vi "test_fpga.vi"() -> ()   [LabVIEW 2014, in "SYSID.lvlib"]
doc: "This VI was generated automatically using the FPGA Wizard. You can modify the VI normally."
uses:
  SYSID.lvlib
  <vilib>/Platform/TimedLoop/XDataNode/timing_clust.ctl
  <vilib>/Platform/TimedLoop/XDataNode/nitl_modes.ctl
  <vilib>/Platform/TimedLoop/XDataNode/wakeup.ctl
  <vilib>/rvi/Emulation/niFpgaGetClockAttributes.vi
  <vilib>/rvi/Emulation/niFpgaSctlEmulationGetInTimedLoop.vi
  <vilib>/rvi/Emulation/niFpgaEmulationReportErrorSimple.vi
  <vilib>/rvi/Emulation/niFpgaProcessEmulError.vi
  <vilib>/rvi/eio/common/nirviEmuTemplateMethod_errors.vi
  <vilib>/rvi/Emulation/niFpgaCriticalErrorInLSC.vi
  <vilib>/eio/EIONode/EIONode.xnode
  <vilib>/Platform/TimedLoop/XDataNode/XDataNode.xnode
  <vilib>/Platform/TimedLoop/XDataNode/XDNodeRunTimeDep.lvlib
panel:
  out "velocity":sgl
  out "Pendulum Position":i32
  out "_Pendulum Position":i32
  in  "Pendulum Reset":bool
  out "Right Limit":bool
  out "Left Limit":bool
  in  "Brake":bool=TRUE
  in  "Amp Reset":bool=TRUE
  in  "Amp Enable":bool
  out "quad saved (Port0/DIO0,Port0/DIO1)":cluster{"Position":i32, "Index Count":u16}
  out "Stage Position":i32
  out "_quad pos (Port0/DIO0,Port0/DIO1)":i32
  in  "quad reset (Port0/DIO0,Port0/DIO1)":bool
  out "_quad saved (Port0/DIO0,Port0/DIO1)":cluster{"Position":i32, "Index Count":u16}
  in  "AO (ModB/AO2)":fxp<+/-,20,5>
  in  "Drive Command":fxp<+/-,20,5>
  out "AI (ModA/AI0)":fxp<+/-,26,5> format="%.6g"
  in  "Local Stop 0":bool
  out "Actual Loop Rate (Ticks)":u32
  out "Late? Latched":bool
  in  "Loop Rate (Ticks)":u32=571
  in  "Reset":bool
  in  "Start 0":bool
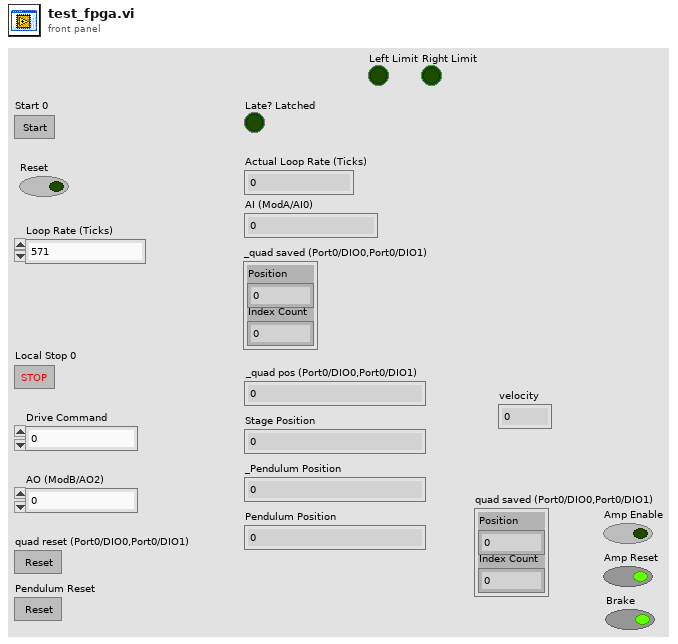
[diagram p1: front panel]
types:
  T1 = typedef "XDNodeRunTimeDep.lvlib/timing_clust.ctl" = cluster{"Expected End [f-1]":u64, "Actual End [f-1]":u64, "Finished Late? [f-1]":bool, "Expected End [i-1]":u64, "Actual End [i-1]":u64, "Finished Late? [i-1]":bool, "Expected Start [i]":u64, "Actual Start [i]":u64, "Expected Start [f]":u64, "Actual Start [f]":u64, "Source Name":string, "Structure Name":string, "Period":i64, "Deadline":i64, "Offset":i64, "Start":i64, "Priority":i32, "Timeout":i32, "Mode":T2, "Wakeup Reason":T3, "Error":errorcluster, "Source Type":string, "Secondary Source Type":string, "Global End Time":u64, "Global Start Time":u64, "Frame Duration":u64, "Iteration Duration":u64, "Assigned CPU":i32, "I/O Scan Engine Mode":u32}
  T2 = typedef "XDNodeRunTimeDep.lvlib/nitl_modes.ctl" = enum32{"No Change", "Process missed periods, maintain original phase", "Discard missed periods, maintain original phase", "Process missed periods, ignore original phase", "Discard missed periods, ignore original phase"}
  T3 = typedef "XDNodeRunTimeDep.lvlib/wakeup.ctl" = enum32{"Normal", "Aborted", "Asynchronous wakeup", "Timing source error", "Timed loop error", "Timeout"}
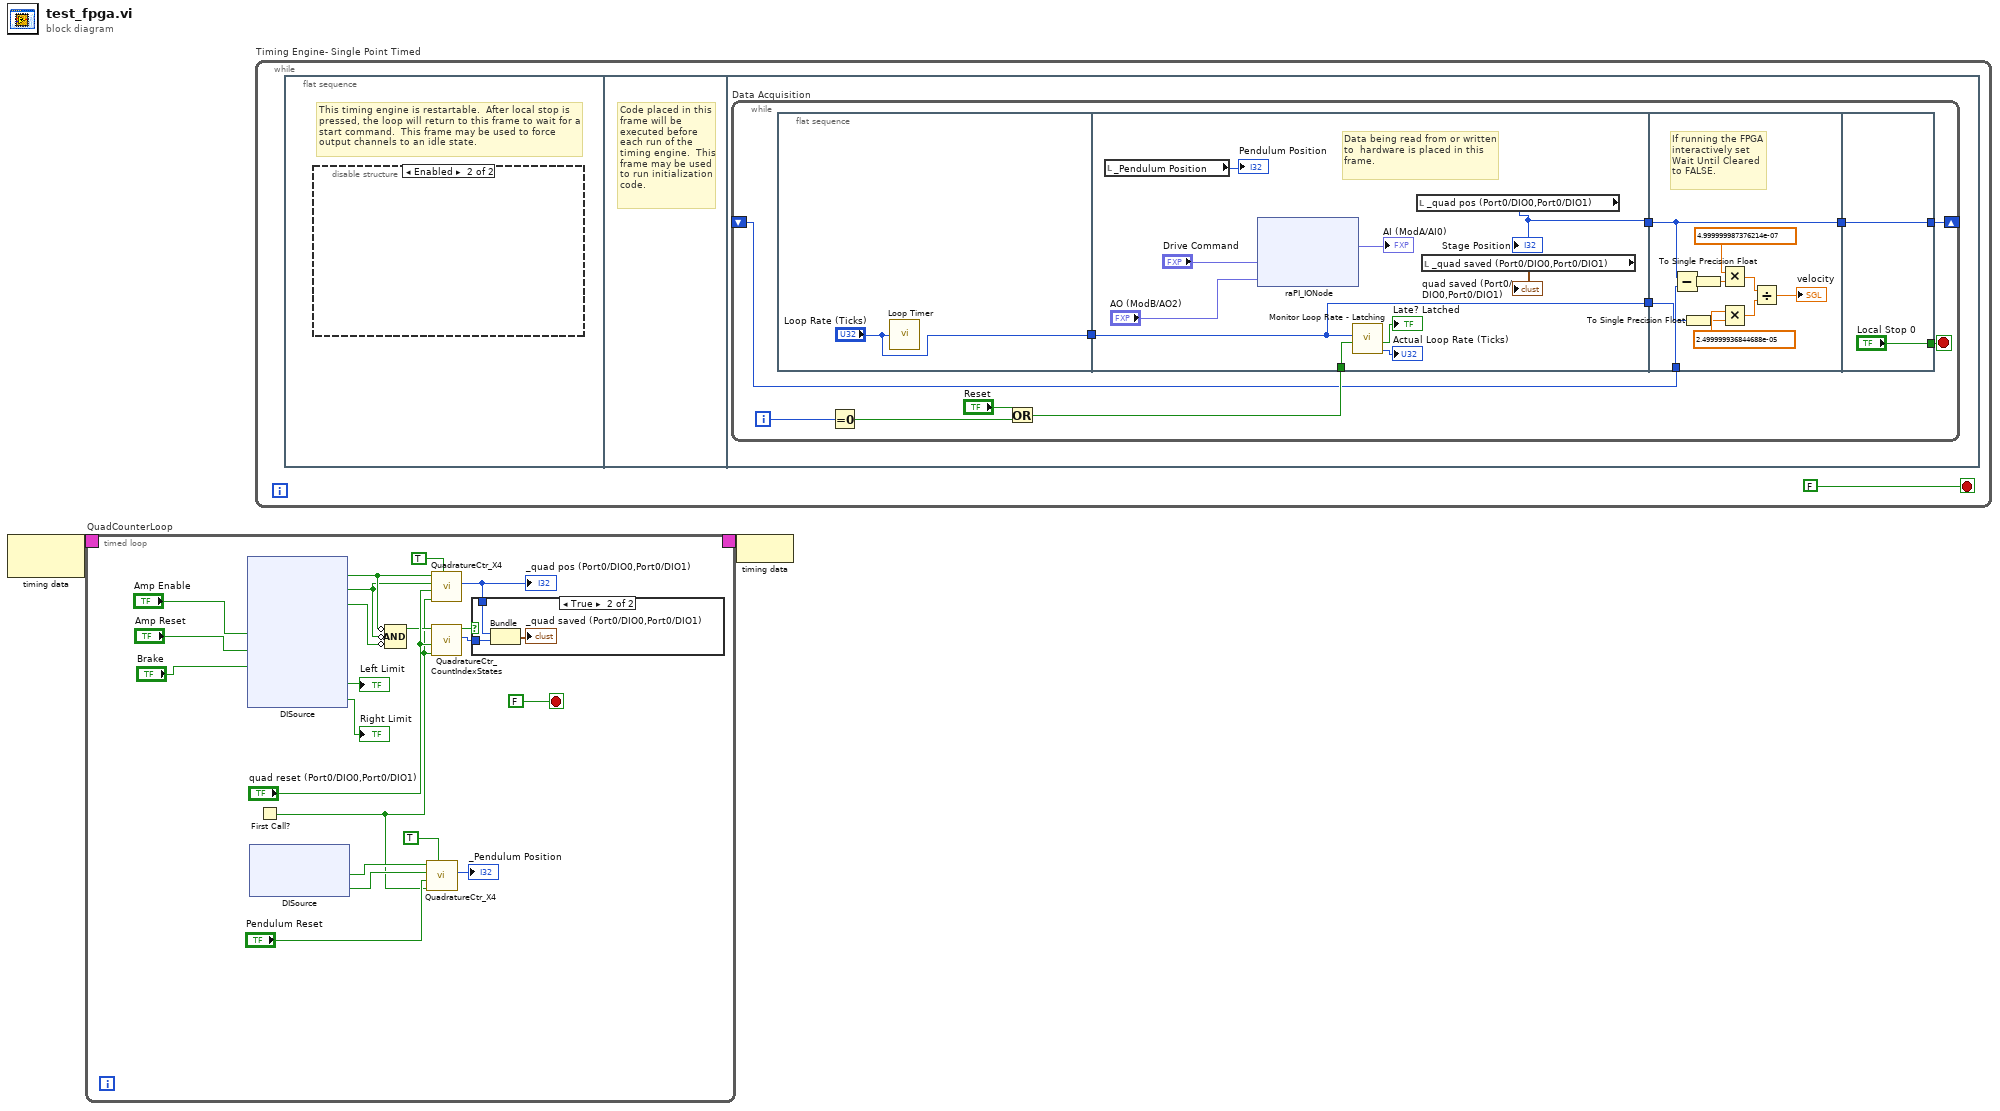
[diagram p0: block diagram]
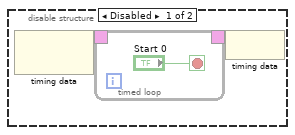
[diagram p3: hidden frame]
diagram:
  n1 = node-c288 ("Input Node")() -> (w2:T1)  [unwired: 1 in]
  n2 = timed-loop "QuadCounterLoop" {
    timing: w2 -> [_]
    timing-out: [_] -> w1
    stop <- FALSE stop-if-true
    n3 = xnode ("DISource")("Port3/DIO4"="Amp Enable", "Port3/DIO8"="Amp Reset", "Port3/DIO3"="Brake") -> ("Port3/DIO0"=w17:bool, "Port3/DIO1"=w16:bool, "Port3/DIO2"=w15:bool, "Port3/DIO5"=→"Left Limit":bool, "Port3/DIO6"=→"Right Limit":bool)  [unwired: 8 in, 8 out]
    n4 = xnode ("DISource")() -> ("Port7/DIO0"=w7:bool, "Port7/DIO1"=w6:bool)  [unwired: 2 in, 2 out]
    n5 = First Call?() -> (First Call?: T/F=w4:bool)
    n6 = Compound Arithmetic op=AND(invert w17, invert w16, invert w15) -> (w14:bool)
    n7 = call "QuadratureCtr_X4.vi"("Direction?"=TRUE, "First Run?"=w4, "Reset"="Pendulum Reset", "Source B"=w6, "Source A"=w7) -> ("Position"=→"_Pendulum Position":i32)  [unwired: 6 in]
    n8 = call "QuadratureCtr_X4.vi"("Direction?"=TRUE, "First Run?"=w4, "Reset"="quad reset (Port0/DIO0,Port0/DIO1)", "Source B"=w16, "Source A"=w17) -> ("Position"=w21:i32)  [unwired: 6 in]
    "_quad pos (Port0/DIO0,Port0/DIO1)" <- w21
    n9 = call "QuadratureCtr_CountIndexStates.vi"("First Run?"=w4, "Reset"="quad reset (Port0/DIO0,Port0/DIO1)", "Valid Index State?"=w14) -> ("Index State Count"=w19:u16, "Save State?"=w18:bool)  [unwired: 7 in]
    n10 = case shown="True" w18 {
      tunnel: w21 -> [_ w26]
      tunnel: w19 -> [_ w24]
      frame False {
      }
      frame True {
        n11 = Bundle("Position"=w26, "Index State Count"=w24) -> (→"_quad saved (Port0/DIO0,Port0/DIO1)":cluster{"Position":i32, "Index State Count":u16})  [unwired: 1 in]
      }
    }
  }
  n12 = while "Timing Engine- Single Point Timed" {
    stop <- FALSE stop-if-true
    n13 = flat-sequence "MainSeq" {
      frame #0 {
        # "This timing engine is restartable.  After local stop is pressed, the loop will return to this frame to wait for a start command.  This frame may be used to force output channels to an idle state."
        n14 = disable-structure shown="Enabled" {
          frame Disabled {
            n15 = node-c288 ("Input Node")() -> (w31:T1)  [unwired: 1 in]
            n16 = timed-loop "initWait" {
              timing: w31 -> [_]
              timing-out: [_] -> w30
              stop <- "Start 0" stop-if-true
            }
            n17 = node-c288 ("Output Node")(w30) -> ()
          }
          frame Enabled {
          }
        }
      }
      frame #1 {
        # "Code placed in this frame will be executed before each run of the timing engine.  This frame may be used to run initialization code."
      }
      frame #2 {
        n18 = while "Data Acquisition" {
          shift-right: [w39] -> _
          shift-left: _ -> [w38]
          i -> [w45]
          stop <- w47 stop-if-true
          n19 = flat-sequence "Data Acquisition Sequence" {
            tunnel: ["Loop Rate (Ticks)"] -> w46
            tunnel: w46 -> [w49]
            tunnel: w42 -> [w56]
            tunnel: [w50] -> w41
            tunnel: [w49] -> w37
            tunnel: w41 -> [w69]
            tunnel: [w69] -> w40
            tunnel: w38 -> [w68]
            tunnel: w37 -> [w64]
            tunnel: ["Local Stop 0"] -> w47
            tunnel: w40 -> [w70]
            tunnel: [w70] -> w39
            frame #0 {
              n20 = call "Loop Timer"("Count(Ticks)"="Loop Rate (Ticks)") -> ()  [unwired: 1 out]
            }
            frame #1 {
              # "Data being read from or written to  hardware is placed in this frame."
              n21 = local read "_Pendulum Position"() -> (→"Pendulum Position":i32)
              n22 = xnode ("raPI_IONode")("ModB/AO0"="Drive Command", "ModB/AO2"="AO (ModB/AO2)") -> ("ModA/AI0"=→"AI (ModA/AI0)":fxp<+/-,26,5>)  [unwired: 3 in, 3 out]
              n23 = call "Monitor Loop Rate - Latching.vi"("Reset"=w56, "Count(Ticks)"=w49) -> ("Actual Loop Rate (Ticks)"=→"Actual Loop Rate (Ticks)":u32, "Late? (Latched)"=→"Late? Latched":bool)  [unwired: 7 in, 1 out]
              n24 = local read "_quad pos (Port0/DIO0,Port0/DIO1)"() -> (w50:i32)
              "Stage Position" <- w50
              n25 = local read "_quad saved (Port0/DIO0,Port0/DIO1)"() -> (→"quad saved (Port0/DIO0,Port0/DIO1)":cluster{"Position":i32, "Index Count":u16})
            }
            frame #2 {
              # "If running the FPGA interactively set Wait Until Cleared to FALSE."
              n26 = Subtract(x=w69, y=w68) -> (x-y=w66:i32)
              n27 = To Single Precision Float(number=w64) -> (single precision float=w60:sgl)
              n28 = To Single Precision Float(number=w66) -> (single precision float=w61:sgl)
              n29 = Multiply(x=sgl 5e-07, y=w61) -> (x*y=w63:sgl)
              n30 = Multiply(x=sgl 2.5e-05, y=w60) -> (x*y=w62:sgl)
              n31 = Divide(x=w63, y=w62) -> (x/y=→"velocity":sgl)
            }
            frame #3 {
            }
          }
          n32 = Equal To 0?(x=w45) -> (x = 0?=w44:bool)
          n33 = Or(x="Reset", y=w44) -> (x .or. y?=w42:bool)
        }
      }
    }
  }
  n34 = node-c288 ("Output Node")(w1) -> ()
